vi "数据发送组合-20200825 (子VI).vi"(10 "枚举":T2(ring), 11 "插值后的数组元素":T1) -> (3 "字符串":string)   [LabVIEW 2016, in "数据传输系统-05.lvlib"]
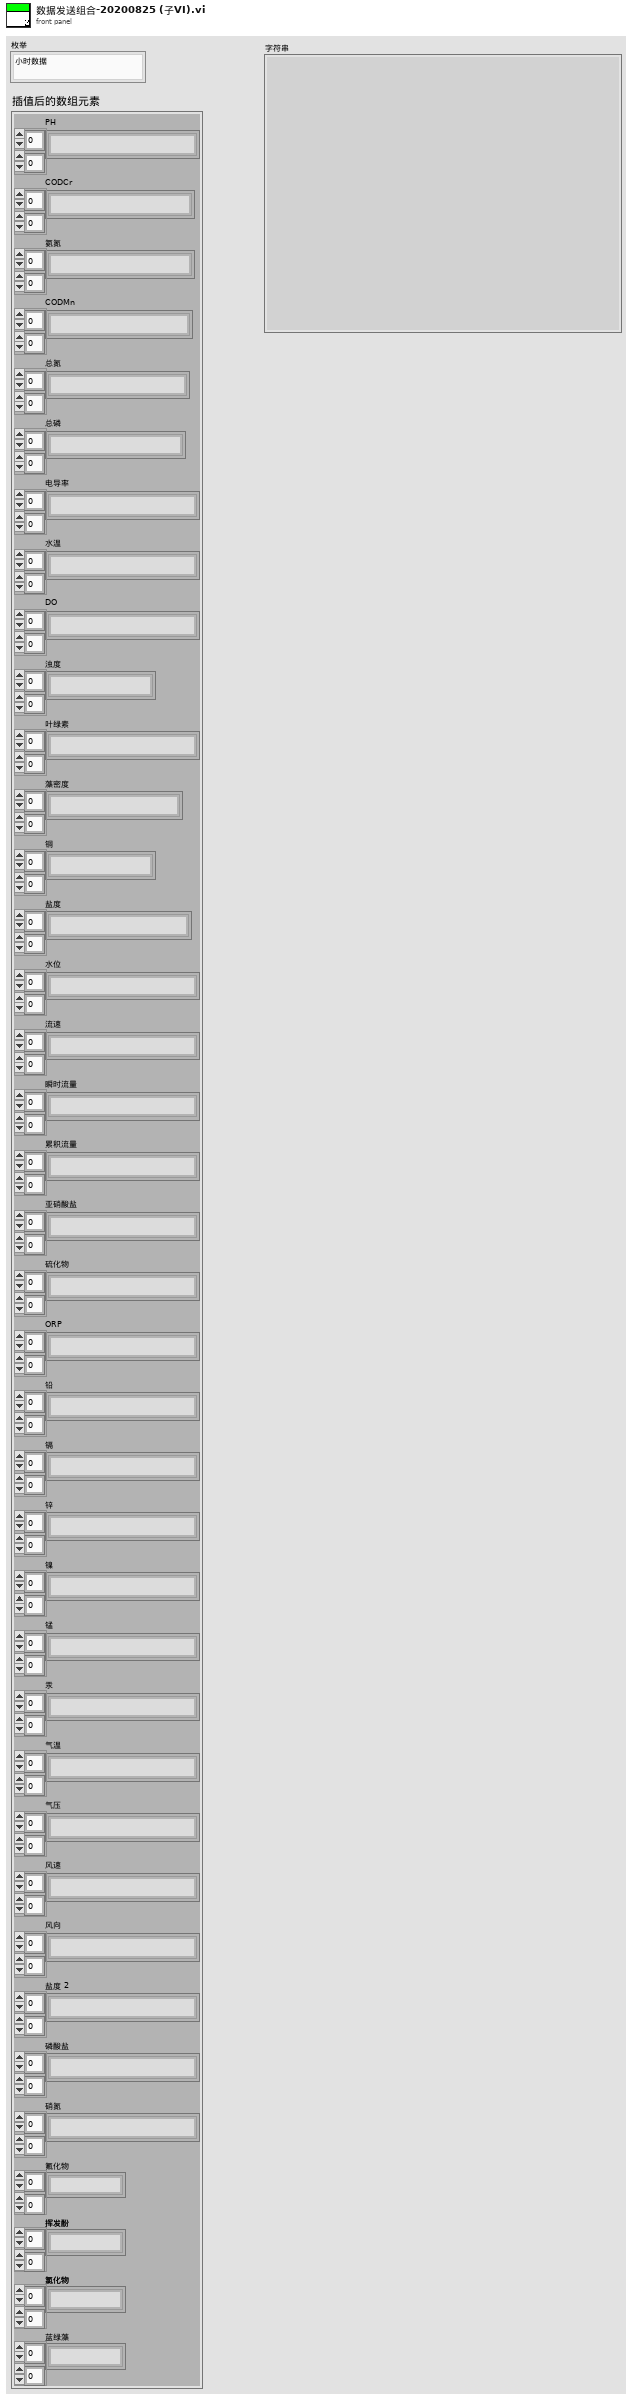
[diagram p1: front panel]
types:
  T1 = cluster{"PH":string[][], "CODCr":string[][], "氨氮":string[][], "CODMn":string[][], "总氮":string[][], "总磷":string[][], "电导率":string[][], "水温":string[][], "DO":string[][], "浊度":string[][], "叶绿素":string[][], "藻密度":string[][], "铜":string[][], "盐度":string[][], "水位":string[][], "流速":string[][], "瞬时流量":string[][], "累积流量":string[][], "亚硝酸盐":string[][], "硫化物":string[][], "ORP":string[][], "铅":string[][], "镉":string[][], "锌":string[][], "镍":string[][], "锰":string[][], "汞":string[][], "气温":string[][], "气压":string[][], "风速":string[][], "风向":string[][], "盐度 2":string[][], "磷酸盐":string[][], "硝氮":string[][], "氟化物":string[][], "挥发酚":string[][], "氯化物":string[][], "蓝绿藻":string[][]}
  T2 = enum16{"小时数据", "实时数据", "平行样测试", "集成干预测试", "加标回收测试", "核查数据", "空白零点跨度数据", "提取小时数据", "提取实时数据", "操作日志", "仪器参数", "3090仪器参数", "提取仪器参数", "报警信息"}
  T3 = cluster{"PH":string[][], "CODCr":string[][], "氨氮":string[][], "CODMn":string[][], "总氮":string[][], "总磷":string[][], "电导率":string[][], "水温":string[][], "DO":string[][], "浊度":string[][], "叶绿素":string[][], "藻密度":string[][], "铜":string[][], "盐度":string[][], "水位":string[][], "流速":string[][], "瞬时流量":string[][], "累积流量":string[][], "亚硝酸盐":string[][], "硫化物":string[][], "ORP":string[][], "铅":string[][], "镉":string[][], "锌":string[][], "镍":string[][], "锰":string[][], "汞":string[][], "气温":string[][], "气压":string[][], "风速":string[][], "风向":string[][], "盐度 2":string[][], "磷酸盐":string[][], "硝氮":string[][], "氟化物":string[][], "挥发酚":string[][], "氯化物":string[][]}
  T4 = cluster{"CODMn":dbl, "CODCr":dbl, "DO":dbl, "铜":dbl, "PH":dbl, "氨氮":dbl, "比电导率":dbl, "水温":dbl, "COD":dbl, "浊度":dbl, "总氮":dbl, "总磷":dbl, "叶绿素a":dbl, "藻密度":dbl, "水位":dbl, "流速":dbl, "瞬时流量":dbl, "累积流量":dbl, "亚硝酸盐":dbl, "硫化物":dbl, "ORP":dbl, "铅":dbl, "镉":dbl, "锌":dbl, "镍":dbl, "锰":dbl, "汞":dbl, "气温":dbl, "气压":dbl, "风速":dbl, "风向":dbl, "盐度":dbl, "磷酸盐":dbl, "硝氮":dbl, "氟化物":dbl, "挥发酚":dbl, "氯化物":dbl, "蓝绿藻":dbl}
  T5 = cluster{"CODMn":string, "CODCr":string, "DO":string, "铜":string, "PH":string, "氨氮":string, "比电导率":string, "水温":string, "COD":string, "浊度":string, "总氮":string, "总磷":string, "叶绿素a":string, "藻密度":string, "水位":string, "流速":string, "瞬时流量":string, "累积流量":string, "亚硝酸盐":string, "硫化物":string, "ORP":string, "铅":string, "镉":string, "锌":string, "镍":string, "锰":string, "汞":string, "气温":string, "气压":string, "风速":string, "风向":string, "盐度":string, "磷酸盐":string, "硝氮":string, "氟化物":string, "挥发酚":string, "氯化物":string, "蓝绿藻":string}
  T6 = typedef "数据传输系统-05.lvlib/应用环境.ctl" = enum16{"STD", "GB212", "婉仪平台"}
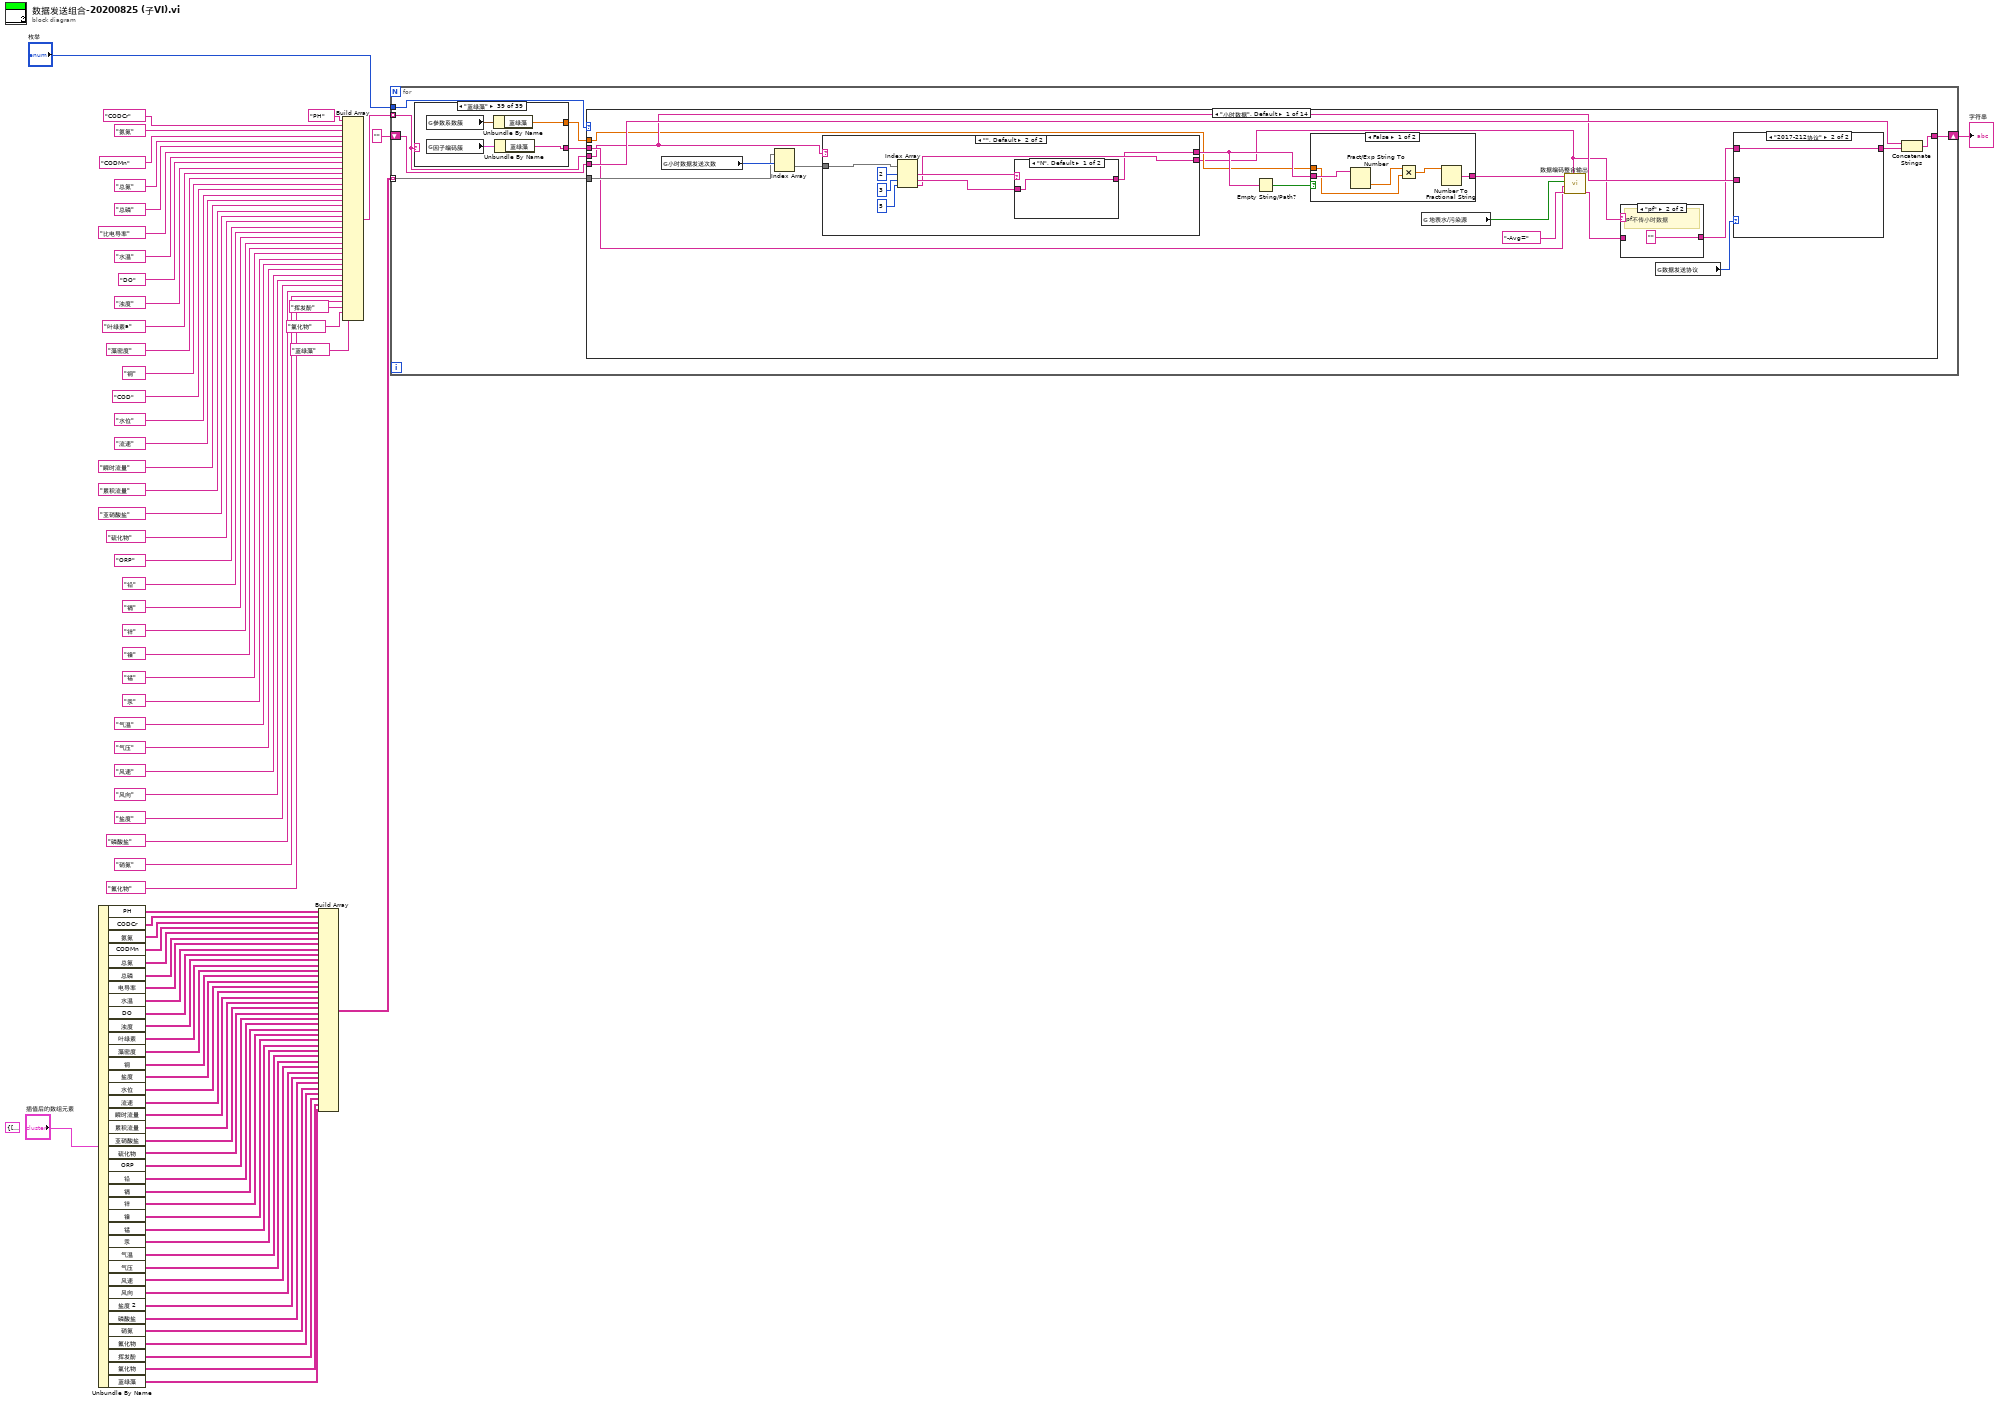
[diagram p0: block diagram]
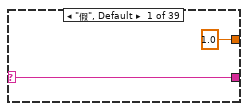
[diagram p2: hidden frame]
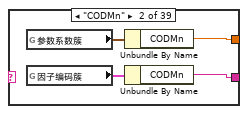
[diagram p3: hidden frame]
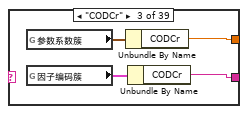
[diagram p4: hidden frame]
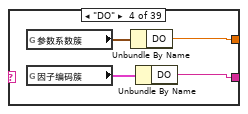
[diagram p5: hidden frame]
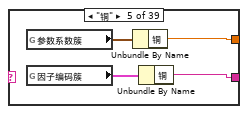
[diagram p6: hidden frame]
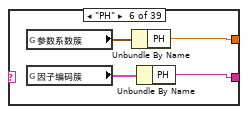
[diagram p7: hidden frame]
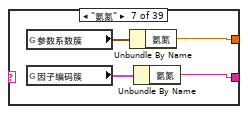
[diagram p8: hidden frame]
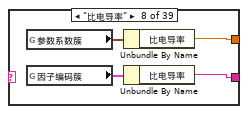
[diagram p9: hidden frame]
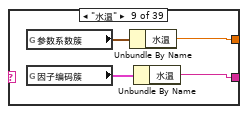
[diagram p10: hidden frame]
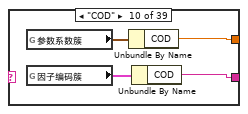
[diagram p11: hidden frame]
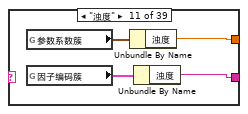
[diagram p12: hidden frame]
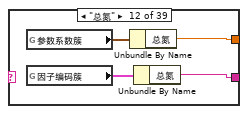
[diagram p13: hidden frame]
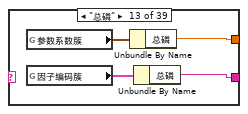
[diagram p14: hidden frame]
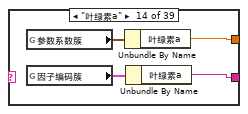
[diagram p15: hidden frame]
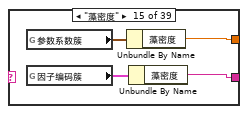
[diagram p16: hidden frame]
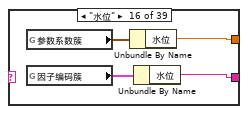
[diagram p17: hidden frame]
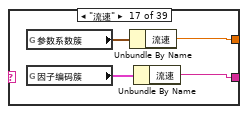
[diagram p18: hidden frame]
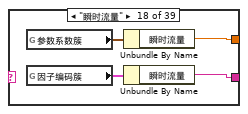
[diagram p19: hidden frame]
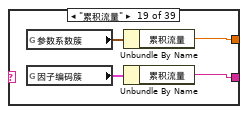
[diagram p20: hidden frame]
diagram:
  (unwired) T3 {"PH"=[], "CODCr"=[], "氨氮"=[], "CODMn"=[], "总氮"=[], "总磷"=[], "电导率"=[], "水温"=[], "DO"=[], "浊度"=[], "叶绿素"=[], "藻密度"=[], "铜"=[], "盐度"=[], "水位"=[], "流速"=[], "瞬时流量"=[], "累积流量"=[], "亚硝酸盐"=[], "硫化物"=[], "ORP"=[], "铅"=[], "镉"=[], "锌"=[], "镍"=[], "锰"=[], "汞"=[], "气温"=[], "气压"=[], "风速"=[], "风向"=[], "盐度 2"=[], "磷酸盐"=[], "硝氮"=[], "氟化物"=[], "挥发酚"=[], "氯化物"=[]} ("插值后的数组元素")
  n1 = Unbundle By Name("插值后的数组元素") -> ("PH"=w82:string[][], "CODCr"=w81:string[][], "氨氮"=w80:string[][], "CODMn"=w79:string[][], "总氮"=w78:string[][], "总磷"=w77:string[][], "电导率"=w76:string[][], "水温"=w75:string[][], "DO"=w74:string[][], "浊度"=w73:string[][], "叶绿素"=w72:string[][], "藻密度"=w71:string[][], "铜"=w70:string[][], "盐度"=w69:string[][], "水位"=w68:string[][], "流速"=w67:string[][], "瞬时流量"=w66:string[][], "累积流量"=w65:string[][], "亚硝酸盐"=w64:string[][], "硫化物"=w63:string[][], "ORP"=w62:string[][], "铅"=w61:string[][], "镉"=w60:string[][], "锌"=w59:string[][], "镍"=w58:string[][], "锰"=w57:string[][], "汞"=w56:string[][], "气温"=w20:string[][], "气压"=w21:string[][], "风速"=w22:string[][], "风向"=w23:string[][], "盐度 2"=w14:string[][], "磷酸盐"=w13:string[][], "硝氮"=w12:string[][], "氟化物"=w8:string[][], "挥发酚"=w6:string[][], "氯化物"=w5:string[][], "蓝绿藻"=w1:string[][])
  n2 = Build Array(w82, w81, w80, w79, w78, w77, w76, w75, w74, w73, w72, w71, w70, w69, w68, w67, w66, w65, w64, w63, w62, w61, w60, w59, w58, w57, w56, w20, w21, w22, w23, w14, w13, w12, w8, w6, w5, w1) -> (w55:string[][][])
  n3 = Build Array("PH" ("污染物编码"), "CODCr" ("污染物编码"), "氨氮" ("污染物编码"), "CODMn" ("污染物编码"), "总氮" ("污染物编码"), "总磷" ("污染物编码"), "比电导率" ("污染物编码"), "水温" ("污染物编码"), "DO" ("污染物编码"), "浊度" ("污染物编码"), "叶绿素a" ("污染物编码"), "藻密度" ("污染物编码"), "铜" ("污染物编码"), "COD" ("污染物编码"), "水位" ("污染物编码"), "流速" ("污染物编码"), "瞬时流量" ("污染物编码"), "累积流量" ("污染物编码"), "亚硝酸盐" ("污染物编码"), "硫化物" ("污染物编码"), "ORP" ("污染物编码"), "铅" ("污染物编码"), "镉" ("污染物编码"), "锌" ("污染物编码"), "镍" ("污染物编码"), "锰" ("污染物编码"), "汞" ("污染物编码"), "气温" ("污染物编码"), "气压" ("污染物编码"), "风速" ("污染物编码"), "风向" ("污染物编码"), "盐度" ("污染物编码"), "磷酸盐" ("污染物编码"), "硝氮" ("污染物编码"), "氟化物" ("污染物编码"), "挥发酚" ("污染物编码"), "氯化物" ("污染物编码"), "蓝绿藻" ("污染物编码")) -> (w27:string[])
  n4 = for {
    tunnel: w55 -> [w89] mode=indexing
    tunnel: w27 -> [w84] mode=indexing
    shift-right: [w88] -> w25
    shift-left: "" -> [w87]
    tunnel: "枚举" -> [w86]
    n5 = case shown="\"蓝绿藻\"" w84 {
      selector: w84 -> [w91 _ _ _ _ _ _ _ _ _ _ _ _ _ _ _ _ _ _ _ _ _ _ _ _ _ _ _ _ _ _ _ _ _ _ _ _ _ _]
      tunnel: [w91 w94 w98 w102 w106 w110 w114 w118 w122 w126 w130 w134 w138 w142 w146 w150 w154 w158 w162 w166 w170 w174 w178 w182 w186 w190 w194 w198 w202 w206 w210 w214 w218 w222 w226 w230 w234 w238 w242] -> w85
      tunnel: [1.0 ("风向") w92 w96 w100 w104 w108 w112 w116 w120 w124 w128 w132 w136 w140 w144 w148 w152 w156 w160 w164 w168 w172 w176 w180 w184 w188 w192 w196 w200 w204 w208 w212 w216 w220 w224 w228 w232 w236 w240] -> w83
      frame "假", Default {
      }
      frame "CODMn" {
        n6 = global read "断电保存全局.vi" "参数系数簇"() -> (w93:T4)
        n7 = global read "断电保存全局.vi" "因子编码簇"() -> (w95:T5)
        n8 = Unbundle By Name(w93) -> ("CODMn"=w92:dbl)
        n9 = Unbundle By Name(w95) -> ("CODMn"=w94:string)
      }
      frame "CODCr" {
        n10 = global read "断电保存全局.vi" "参数系数簇"() -> (w97:T4)
        n11 = global read "断电保存全局.vi" "因子编码簇"() -> (w99:T5)
        n12 = Unbundle By Name(w97) -> ("CODCr"=w96:dbl)
        n13 = Unbundle By Name(w99) -> ("CODCr"=w98:string)
      }
      frame "DO" {
        n14 = global read "断电保存全局.vi" "参数系数簇"() -> (w101:T4)
        n15 = global read "断电保存全局.vi" "因子编码簇"() -> (w103:T5)
        n16 = Unbundle By Name(w101) -> ("DO"=w100:dbl)
        n17 = Unbundle By Name(w103) -> ("DO"=w102:string)
      }
      frame "铜" {
        n18 = global read "断电保存全局.vi" "参数系数簇"() -> (w105:T4)
        n19 = global read "断电保存全局.vi" "因子编码簇"() -> (w107:T5)
        n20 = Unbundle By Name(w105) -> ("铜"=w104:dbl)
        n21 = Unbundle By Name(w107) -> ("铜"=w106:string)
      }
      frame "PH" {
        n22 = global read "断电保存全局.vi" "参数系数簇"() -> (w109:T4)
        n23 = global read "断电保存全局.vi" "因子编码簇"() -> (w111:T5)
        n24 = Unbundle By Name(w109) -> ("PH"=w108:dbl)
        n25 = Unbundle By Name(w111) -> ("PH"=w110:string)
      }
      frame "氨氮" {
        n26 = global read "断电保存全局.vi" "参数系数簇"() -> (w113:T4)
        n27 = global read "断电保存全局.vi" "因子编码簇"() -> (w115:T5)
        n28 = Unbundle By Name(w113) -> ("氨氮"=w112:dbl)
        n29 = Unbundle By Name(w115) -> ("氨氮"=w114:string)
      }
      frame "比电导率" {
        n30 = global read "断电保存全局.vi" "参数系数簇"() -> (w117:T4)
        n31 = global read "断电保存全局.vi" "因子编码簇"() -> (w119:T5)
        n32 = Unbundle By Name(w117) -> ("比电导率"=w116:dbl)
        n33 = Unbundle By Name(w119) -> ("比电导率"=w118:string)
      }
      frame "水温" {
        n34 = global read "断电保存全局.vi" "参数系数簇"() -> (w121:T4)
        n35 = global read "断电保存全局.vi" "因子编码簇"() -> (w123:T5)
        n36 = Unbundle By Name(w121) -> ("水温"=w120:dbl)
        n37 = Unbundle By Name(w123) -> ("水温"=w122:string)
      }
      frame "COD" {
        n38 = global read "断电保存全局.vi" "参数系数簇"() -> (w125:T4)
        n39 = global read "断电保存全局.vi" "因子编码簇"() -> (w127:T5)
        n40 = Unbundle By Name(w125) -> ("COD"=w124:dbl)
        n41 = Unbundle By Name(w127) -> ("COD"=w126:string)
      }
      frame "浊度" {
        n42 = global read "断电保存全局.vi" "参数系数簇"() -> (w129:T4)
        n43 = global read "断电保存全局.vi" "因子编码簇"() -> (w131:T5)
        n44 = Unbundle By Name(w129) -> ("浊度"=w128:dbl)
        n45 = Unbundle By Name(w131) -> ("浊度"=w130:string)
      }
      frame "总氮" {
        n46 = global read "断电保存全局.vi" "参数系数簇"() -> (w133:T4)
        n47 = global read "断电保存全局.vi" "因子编码簇"() -> (w135:T5)
        n48 = Unbundle By Name(w133) -> ("总氮"=w132:dbl)
        n49 = Unbundle By Name(w135) -> ("总氮"=w134:string)
      }
      frame "总磷" {
        n50 = global read "断电保存全局.vi" "参数系数簇"() -> (w137:T4)
        n51 = global read "断电保存全局.vi" "因子编码簇"() -> (w139:T5)
        n52 = Unbundle By Name(w137) -> ("总磷"=w136:dbl)
        n53 = Unbundle By Name(w139) -> ("总磷"=w138:string)
      }
      frame "叶绿素a" {
        n54 = global read "断电保存全局.vi" "参数系数簇"() -> (w141:T4)
        n55 = global read "断电保存全局.vi" "因子编码簇"() -> (w143:T5)
        n56 = Unbundle By Name(w141) -> ("叶绿素a"=w140:dbl)
        n57 = Unbundle By Name(w143) -> ("叶绿素a"=w142:string)
      }
      frame "藻密度" {
        n58 = global read "断电保存全局.vi" "参数系数簇"() -> (w145:T4)
        n59 = global read "断电保存全局.vi" "因子编码簇"() -> (w147:T5)
        n60 = Unbundle By Name(w145) -> ("藻密度"=w144:dbl)
        n61 = Unbundle By Name(w147) -> ("藻密度"=w146:string)
      }
      frame "水位" {
        n62 = global read "断电保存全局.vi" "参数系数簇"() -> (w149:T4)
        n63 = global read "断电保存全局.vi" "因子编码簇"() -> (w151:T5)
        n64 = Unbundle By Name(w149) -> ("水位"=w148:dbl)
        n65 = Unbundle By Name(w151) -> ("水位"=w150:string)
      }
      frame "流速" {
        n66 = global read "断电保存全局.vi" "参数系数簇"() -> (w153:T4)
        n67 = global read "断电保存全局.vi" "因子编码簇"() -> (w155:T5)
        n68 = Unbundle By Name(w153) -> ("流速"=w152:dbl)
        n69 = Unbundle By Name(w155) -> ("流速"=w154:string)
      }
      frame "瞬时流量" {
        n70 = global read "断电保存全局.vi" "参数系数簇"() -> (w157:T4)
        n71 = global read "断电保存全局.vi" "因子编码簇"() -> (w159:T5)
        n72 = Unbundle By Name(w157) -> ("瞬时流量"=w156:dbl)
        n73 = Unbundle By Name(w159) -> ("瞬时流量"=w158:string)
      }
      frame "累积流量" {
        n74 = global read "断电保存全局.vi" "参数系数簇"() -> (w161:T4)
        n75 = global read "断电保存全局.vi" "因子编码簇"() -> (w163:T5)
        n76 = Unbundle By Name(w161) -> ("累积流量"=w160:dbl)
        n77 = Unbundle By Name(w163) -> ("累积流量"=w162:string)
      }
      frame "亚硝酸盐" {
        n78 = global read "断电保存全局.vi" "参数系数簇"() -> (w165:T4)
        n79 = global read "断电保存全局.vi" "因子编码簇"() -> (w167:T5)
        n80 = Unbundle By Name(w165) -> ("亚硝酸盐"=w164:dbl)
        n81 = Unbundle By Name(w167) -> ("亚硝酸盐"=w166:string)
      }
      frame "硫化物" {
        n82 = global read "断电保存全局.vi" "参数系数簇"() -> (w169:T4)
        n83 = global read "断电保存全局.vi" "因子编码簇"() -> (w171:T5)
        n84 = Unbundle By Name(w169) -> ("硫化物"=w168:dbl)
        n85 = Unbundle By Name(w171) -> ("硫化物"=w170:string)
      }
      frame "ORP" {
        n86 = global read "断电保存全局.vi" "参数系数簇"() -> (w173:T4)
        n87 = global read "断电保存全局.vi" "因子编码簇"() -> (w175:T5)
        n88 = Unbundle By Name(w173) -> ("ORP"=w172:dbl)
        n89 = Unbundle By Name(w175) -> ("ORP"=w174:string)
      }
      frame "铅" {
        n90 = global read "断电保存全局.vi" "参数系数簇"() -> (w177:T4)
        n91 = global read "断电保存全局.vi" "因子编码簇"() -> (w179:T5)
        n92 = Unbundle By Name(w177) -> ("铅"=w176:dbl)
        n93 = Unbundle By Name(w179) -> ("铅"=w178:string)
      }
      frame "镉" {
        n94 = global read "断电保存全局.vi" "参数系数簇"() -> (w181:T4)
        n95 = global read "断电保存全局.vi" "因子编码簇"() -> (w183:T5)
        n96 = Unbundle By Name(w181) -> ("镉"=w180:dbl)
        n97 = Unbundle By Name(w183) -> ("镉"=w182:string)
      }
      frame "锌" {
        n98 = global read "断电保存全局.vi" "参数系数簇"() -> (w185:T4)
        n99 = global read "断电保存全局.vi" "因子编码簇"() -> (w187:T5)
        n100 = Unbundle By Name(w185) -> ("锌"=w184:dbl)
        n101 = Unbundle By Name(w187) -> ("锌"=w186:string)
      }
      frame "镍" {
        n102 = global read "断电保存全局.vi" "参数系数簇"() -> (w189:T4)
        n103 = global read "断电保存全局.vi" "因子编码簇"() -> (w191:T5)
        n104 = Unbundle By Name(w189) -> ("镍"=w188:dbl)
        n105 = Unbundle By Name(w191) -> ("镍"=w190:string)
      }
      frame "锰" {
        n106 = global read "断电保存全局.vi" "参数系数簇"() -> (w193:T4)
        n107 = global read "断电保存全局.vi" "因子编码簇"() -> (w195:T5)
        n108 = Unbundle By Name(w193) -> ("锰"=w192:dbl)
        n109 = Unbundle By Name(w195) -> ("锰"=w194:string)
      }
      frame "汞" {
        n110 = global read "断电保存全局.vi" "参数系数簇"() -> (w197:T4)
        n111 = global read "断电保存全局.vi" "因子编码簇"() -> (w199:T5)
        n112 = Unbundle By Name(w197) -> ("汞"=w196:dbl)
        n113 = Unbundle By Name(w199) -> ("汞"=w198:string)
      }
      frame "气温" {
        n114 = global read "断电保存全局.vi" "参数系数簇"() -> (w201:T4)
        n115 = global read "断电保存全局.vi" "因子编码簇"() -> (w203:T5)
        n116 = Unbundle By Name(w201) -> ("气温"=w200:dbl)
        n117 = Unbundle By Name(w203) -> ("气温"=w202:string)
      }
      frame "气压" {
        n118 = global read "断电保存全局.vi" "参数系数簇"() -> (w205:T4)
        n119 = global read "断电保存全局.vi" "因子编码簇"() -> (w207:T5)
        n120 = Unbundle By Name(w205) -> ("气压"=w204:dbl)
        n121 = Unbundle By Name(w207) -> ("气压"=w206:string)
      }
      frame "风速" {
        n122 = global read "断电保存全局.vi" "参数系数簇"() -> (w209:T4)
        n123 = global read "断电保存全局.vi" "因子编码簇"() -> (w211:T5)
        n124 = Unbundle By Name(w209) -> ("风速"=w208:dbl)
        n125 = Unbundle By Name(w211) -> ("风速"=w210:string)
      }
      frame "风向" {
        n126 = global read "断电保存全局.vi" "参数系数簇"() -> (w213:T4)
        n127 = global read "断电保存全局.vi" "因子编码簇"() -> (w215:T5)
        n128 = Unbundle By Name(w213) -> ("风向"=w212:dbl)
        n129 = Unbundle By Name(w215) -> ("风向"=w214:string)
      }
      frame "盐度" {
        n130 = global read "断电保存全局.vi" "参数系数簇"() -> (w217:T4)
        n131 = global read "断电保存全局.vi" "因子编码簇"() -> (w219:T5)
        n132 = Unbundle By Name(w217) -> ("盐度"=w216:dbl)
        n133 = Unbundle By Name(w219) -> ("盐度"=w218:string)
      }
      frame "磷酸盐" {
        n134 = global read "断电保存全局.vi" "参数系数簇"() -> (w221:T4)
        n135 = global read "断电保存全局.vi" "因子编码簇"() -> (w223:T5)
        n136 = Unbundle By Name(w221) -> ("磷酸盐"=w220:dbl)
        n137 = Unbundle By Name(w223) -> ("磷酸盐"=w222:string)
      }
      frame "硝氮" {
        n138 = global read "断电保存全局.vi" "参数系数簇"() -> (w225:T4)
        n139 = global read "断电保存全局.vi" "因子编码簇"() -> (w227:T5)
        n140 = Unbundle By Name(w225) -> ("硝氮"=w224:dbl)
        n141 = Unbundle By Name(w227) -> ("硝氮"=w226:string)
      }
      frame "氟化物" {
        n142 = global read "断电保存全局.vi" "参数系数簇"() -> (w229:T4)
        n143 = global read "断电保存全局.vi" "因子编码簇"() -> (w231:T5)
        n144 = Unbundle By Name(w229) -> ("氟化物"=w228:dbl)
        n145 = Unbundle By Name(w231) -> ("氟化物"=w230:string)
      }
      frame "挥发酚" {
        n146 = global read "断电保存全局.vi" "参数系数簇"() -> (w233:T4)
        n147 = global read "断电保存全局.vi" "因子编码簇"() -> (w235:T5)
        n148 = Unbundle By Name(w233) -> ("挥发酚"=w232:dbl)
        n149 = Unbundle By Name(w235) -> ("挥发酚"=w234:string)
      }
      frame "氯化物" {
        n150 = global read "断电保存全局.vi" "参数系数簇"() -> (w237:T4)
        n151 = global read "断电保存全局.vi" "因子编码簇"() -> (w239:T5)
        n152 = Unbundle By Name(w237) -> ("氯化物"=w236:dbl)
        n153 = Unbundle By Name(w239) -> ("氯化物"=w238:string)
      }
      frame "蓝绿藻" {
        n154 = global read "断电保存全局.vi" "参数系数簇"() -> (w241:T4)
        n155 = global read "断电保存全局.vi" "因子编码簇"() -> (w243:T5)
        n156 = Unbundle By Name(w241) -> ("蓝绿藻"=w240:dbl)
        n157 = Unbundle By Name(w243) -> ("蓝绿藻"=w242:string)
      }
    }
    n158 = case shown="\"小时数据\", Default" w86 {
      tunnel: w89 -> [w258 w303 w334 w343 w398 w404 w416 w440 w462 w499 w517 w524 w534 w556]
      tunnel: w85 -> [w254 w296 w333 w344 w394 w403 w415 w434 w461 w487 w515 w522 w533 w559]
      tunnel: [w257 w300 w335 w341 w399 w400 w412 w431 w460 w494 w512 w521 w529 w545] -> w88
      tunnel: w87 -> [w256 w301 w337 w342 w395 w402 w413 w432 w463 w495 w513 w523 w530 w540]
      tunnel: w84 -> [w252 w295 _ w338 _ _ _ _ _ _ _ _ _ w554]
      tunnel: w83 -> [w249 w291 _ w339 _ _ _ w427 w456 _ _ _ _ _]
      frame "小时数据", Default {
        n159 = global read "全局 小时数据发送次数.vi" "小时数据发送次数"() -> (w261:i32)
        n160 = Index Array(array=w258, index (row)=w261) -> (element=w260:string[])  [unwired: 1 in]
        n161 = case shown="\"\", Default" w252 {
          tunnel: w260 -> [w273 w276]
          tunnel: [w270 w274] -> w250
          tunnel: ["N" ("字符串") w275] -> w246
          frame "风速", "风向", "累积流量", "流速", "气温", "气压", "水位", "瞬时流量" {
            n162 = Index Array(array=w273, index=1 ("索引")) -> (element=w270:string)
          }
          frame "", Default {
            n163 = Index Array(array=w276, index #1=2 ("索引"), index #2=3 ("索引"), index #3=5 ("索引")) -> (element #1=w279:string, element #2=w278:string, element #3=w275:string)
            n164 = case shown="\"N\", Default" w279 {
              tunnel: [w282 ""] -> w274
              tunnel: w278 -> [w282 _]
              frame "N", Default {
              }
              frame "M" {
              }
            }
          }
        }
        n165 = Empty String/Path?(string/path=w250) -> (empty?=w251:bool)
        n166 = case shown="False" w251 {
          tunnel: w250 -> [w267 w269]
          tunnel: w249 -> [w266 _]
          tunnel: [w264 w269] -> w248
          frame False {
            n167 = Fract/Exp String To Number(string=w267) -> (number=w268:dbl)  [unwired: 3 in, 1 out]
            n168 = Multiply(x=w268, y=w266) -> (x*y=w265:dbl)
            n169 = Number To Fractional String(number=w265) -> (F-format string=w264:string)  [unwired: 3 in]
          }
          frame True {
            # "空"
          }
        }
        n170 = global read "断电保存全局.vi" "地表水/污染源"() -> (w247:bool)
        n171 = call "数据编码整合输出.vi"("数据标识"=w246, "数据类型"="-Avg=", "污染物编码"=w254, "地表水/污染源"=w247, "数据值"=w248) -> ("编码输出"=w245:string)  [unwired: 6 in]
        n172 = case shown="\"pf\"" w246 {
          tunnel: w245 -> [w262 _]
          tunnel: [w262 ""] -> w244
          frame "假", Default {
          }
          frame "pf" {
            # "pf不传小时数据"
          }
        }
        n173 = global read "断电保存全局.vi" "数据发送协议"() -> (w255:enum16{"2005-212协议", "2017-212协议"})
        n174 = case shown="\"2017-212协议\"" w255 {
          tunnel: w252 -> [w286 _]
          tunnel: w244 -> [w284 w289]
          tunnel: [w285 w289] -> w253
          frame "2005-212协议", Default {
            n175 = case shown="\"风速\", \"风向\", \"累积流量\", \"流速\", \"气温\", \"气压\", \"水位\"" w286 {
              tunnel: [w287 ""] -> w285
              tunnel: w284 -> [w287 _]
              frame "假", Default {
              }
              frame "风速", "风向", "累积流量", "流速", "气温", "气压", "水位" {
              }
            }
          }
          frame "2017-212协议" {
          }
        }
        n176 = Concatenate Strings(w256, w253) -> (w257:string)
      }
      frame "实时数据" {
        n177 = global read "全局 小时数据发送次数.vi" "小时数据发送次数"() -> (w304:i32)
        n178 = Index Array(array=w303, index (row)=w304) -> (element=w305:string[])  [unwired: 1 in]
        n179 = case shown="\"\", Default" w295 {
          tunnel: w305 -> [w314 w318 w324]
          tunnel: [w313 w317 w323] -> w293
          tunnel: ["N" ("字符串") "N" ("字符串") w321] -> w302
          frame "累积流量", "流速", "水位", "瞬时流量" {
            n180 = Index Array(array=w314, index=1 ("索引")) -> (element=w313:string)
          }
          frame "风速", "风向", "气温", "气压" {
            n181 = Index Array(array=w318, index=1 ("索引")) -> (element=w317:string)
          }
          frame "", Default {
            n182 = Index Array(array=w324, index #1=3 ("索引"), index #2=5 ("索引")) -> (element #1=w323:string, element #2=w321:string)
          }
        }
        n183 = Empty String/Path?(string/path=w293) -> (empty?=w294:bool)
        n184 = case shown="False" w294 {
          tunnel: w293 -> [w310 w312]
          tunnel: w291 -> [w309 _]
          tunnel: [w307 w312] -> w292
          frame False {
            n185 = Fract/Exp String To Number(string=w310) -> (number=w311:dbl)  [unwired: 3 in, 1 out]
            n186 = Multiply(x=w311, y=w309) -> (x*y=w308:dbl)
            n187 = Number To Fractional String(number=w308) -> (F-format string=w307:string)  [unwired: 3 in]
          }
          frame True {
            # "空"
          }
        }
        n188 = global read "断电保存全局.vi" "数据发送协议"() -> (w299:enum16{"2005-212协议", "2017-212协议"})
        n189 = call "数据编码整合输出.vi"("数据标识"=w302, "数据类型"="-Rtd=", "污染物编码"=w296, "地表水/污染源"=FALSE, "数据值"=w292) -> ("编码输出"=w298:string)  [unwired: 6 in]
        n190 = case shown="\"2017-212协议\"" w299 {
          tunnel: w295 -> [w328 _]
          tunnel: w298 -> [w326 w331]
          tunnel: [w327 w331] -> w297
          frame "2005-212协议", Default {
            n191 = case shown="\"假\", Default" w328 {
              tunnel: [w329 ""] -> w327
              tunnel: w326 -> [w329 _]
              frame "假", Default {
              }
              frame "风速", "风向", "累积流量", "流速", "气温", "气压", "水位" {
              }
            }
          }
          frame "2017-212协议" {
          }
        }
        n192 = Concatenate Strings(w301, w297) -> (w300:string)
      }
      frame "平行样测试" {
        n193 = global read "全局 小时数据发送次数.vi" "小时数据发送次数"() -> (w332:i32)
        n194 = call "平行样集成干预数据组合(子VI).vi"("污染物编码"=w333, "数据输入"=w334, "小时数据发送次数"=w332) -> ("输出组合"=w336:string)  [unwired: 8 in]
        n195 = Concatenate Strings(w337, w336) -> (w335:string)
      }
      frame "集成干预测试" {
        n196 = global read "断电保存全局.vi" "应用环境"() -> (w340:T6)
        n197 = case shown="\"GB212\", Default" w340 {
          tunnel: w344 -> [w348 w354]
          tunnel: w343 -> [w347 w355]
          tunnel: w342 -> [w346 w356]
          tunnel: [w345 w351] -> w341
          tunnel: w339 -> [_ w353]
          tunnel: w338 -> [_ w352]
          frame "STD" {
            n198 = global read "全局 小时数据发送次数.vi" "小时数据发送次数"() -> (w349:i32)
            n199 = call "平行样集成干预数据组合(子VI).vi"("污染物编码"=w348, "数据输入"=w347, "小时数据发送次数"=w349) -> ("输出组合"=w350:string)  [unwired: 8 in]
            n200 = Concatenate Strings(w346, w350) -> (w345:string)
          }
          frame "GB212", Default {
            n201 = global read "全局 小时数据发送次数.vi" "小时数据发送次数"() -> (w367:i32)
            n202 = Index Array(array=w355, index (row)=w367) -> (element=w366:string[])  [unwired: 1 in]
            n203 = case shown="\"\", Default" w352 {
              tunnel: w366 -> [w377 w380]
              tunnel: [w374 w379] -> w359
              tunnel: ["N" ("字符串") w378] -> w364
              frame "风速", "风向", "累积流量", "流速", "气温", "气压", "水位", "瞬时流量" {
                n204 = Index Array(array=w377, index=1 ("索引")) -> (element=w374:string)
              }
              frame "", Default {
                n205 = Index Array(array=w380, index #1=2 ("索引"), index #2=3 ("索引"), index #3=5 ("索引")) -> (element #1=w383:string, element #2=w382:string, element #3=w378:string)
                n206 = case shown="\"N\", Default" w383 {
                  tunnel: [w386 ""] -> w379
                  tunnel: w382 -> [w386 _]
                  frame "N", Default {
                  }
                  frame "M" {
                  }
                }
              }
            }
            n207 = Empty String/Path?(string/path=w359) -> (empty?=w360:bool)
            n208 = case shown="False" w360 {
              tunnel: w359 -> [w371 w373]
              tunnel: w353 -> [w370 _]
              tunnel: [w368 w373] -> w358
              frame False {
                n209 = Fract/Exp String To Number(string=w371) -> (number=w372:dbl)  [unwired: 3 in, 1 out]
                n210 = Multiply(x=w372, y=w370) -> (x*y=w369:dbl)
                n211 = Number To Fractional String(number=w369) -> (F-format string=w368:string)  [unwired: 3 in]
              }
              frame True {
                # "空"
              }
            }
            n212 = global read "断电保存全局.vi" "地表水/污染源"() -> (w357:bool)
            n213 = global read "断电保存全局.vi" "数据发送协议"() -> (w363:enum16{"2005-212协议", "2017-212协议"})
            n214 = call "数据编码整合输出.vi"("数据标识"=w364, "数据类型"="-Avg=", "污染物编码"=w354, "地表水/污染源"=w357, "数据值"=w358) -> ("编码输出"=w362:string)  [unwired: 6 in]
            n215 = case shown="\"2017-212协议\"" w363 {
              tunnel: w352 -> [w390 _]
              tunnel: w362 -> [w388 w393]
              tunnel: [w389 w393] -> w361
              frame "2005-212协议", Default {
                n216 = case shown="\"假\", Default" w390 {
                  tunnel: [w391 ""] -> w389
                  tunnel: w388 -> [w391 _]
                  frame "假", Default {
                  }
                  frame "风速", "风向", "累积流量", "流速", "气温", "气压", "水位" {
                  }
                }
              }
              frame "2017-212协议" {
              }
            }
            n217 = Concatenate Strings(w356, w361) -> (w351:string)
          }
        }
      }
      frame "加标回收测试" {
        n218 = global read "全局 小时数据发送次数.vi" "小时数据发送次数"() -> (w397:i32)
        n219 = call "加标回收数据组合 (子VI).vi"("小时数据发送次数"=w397, "数据"=w398, "污染物编码"=w394) -> ("组合输出"=w396:string)  [unwired: 7 in, 1 out]
        n220 = Concatenate Strings(w395, w396) -> (w399:string)
      }
      frame "核查数据" {
        n221 = global read "全局 小时数据发送次数.vi" "小时数据发送次数"() -> (w405:i32)
        n222 = call "标样核查数据组合(子VI).vi"("小时数据发送次数"=w405, "数据输入"=w404, "污染物编码"=w403) -> ("输出组合"=w401:string)  [unwired: 8 in]
        n223 = Concatenate Strings(w402, w401) -> (w400:string)
      }
      frame "空白零点跨度数据" {
        n224 = global read "全局 小时数据发送次数.vi" "小时数据发送次数"() -> (w418:i32)
        n225 = Index Array(array=w416, index (row)=w418) -> (element=w422:string[])  [unwired: 1 in]
        n226 = Index Array(array=w422, index #1=0 ("索引"), index #2=3 ("索引"), index #3=6 ("索引"), index #4=7 ("索引"), index #5=5 ("索引")) -> (element #2=w417:string, element #3=w419:string, element #4=w408:string, element #5=w406:string)  [unwired: 1 out]
        n227 = Empty String/Path?(string/path=w408) -> (empty?=w410:bool)
        n228 = case shown="False" w410 {
          tunnel: [w424 "0" ("span value")] -> w409
          tunnel: w408 -> [w424 _]
          frame False {
          }
          frame True {
          }
        }
        n229 = call "零点跨度数据组合 (子VI).vi"("数据标识"=w406, "span value"=w409, "standard value"=w419, "check value"=w417, "污染物编码"=w415) -> ("组合输出"=w414:string)  [unwired: 6 in]
        n230 = Concatenate Strings(w413, w414) -> (w412:string)
      }
      frame "提取小时数据" {
        n231 = global read "全局 小时数据发送次数.vi" "小时数据发送次数"() -> (w441:i32)
        n232 = Index Array(array=w440, index (row)=w441) -> (element=w439:string[])  [unwired: 1 in]
        n233 = Index Array(array=w439, index #2=1 ("索引")) -> (element #2=w428:string)  [unwired: 1 in, 1 out]
        n234 = Empty String/Path?(string/path=w428) -> (empty?=w430:bool)
        n235 = case shown="False" w430 {
          tunnel: w428 -> [w446 w448]
          tunnel: w427 -> [w445 _]
          tunnel: [w443 w448] -> w429
          frame False {
            n236 = Fract/Exp String To Number(string=w446) -> (number=w447:dbl)  [unwired: 3 in, 1 out]
            n237 = Multiply(x=w447, y=w445) -> (x*y=w444:dbl)
            n238 = Number To Fractional String(number=w444) -> (F-format string=w443:string)  [unwired: 3 in]
          }
          frame True {
            # "空"
          }
        }
        n239 = global read "断电保存全局.vi" "地表水/污染源"() -> (w426:bool)
        n240 = global read "断电保存全局.vi" "数据发送协议"() -> (w436:enum16{"2005-212协议", "2017-212协议"})
        n241 = call "数据编码整合输出.vi"("数据标识"="N", "数据类型"="-Avg=", "污染物编码"=w434, "地表水/污染源"=w426, "数据值"=w429) -> ("编码输出"=w433:string)  [unwired: 6 in]
        n242 = case shown="\"2005-212协议\", Default" w436 {
          tunnel: w434 -> [w451 _]
          tunnel: w433 -> [w449 w454]
          tunnel: [w450 w454] -> w435
          frame "2005-212协议", Default {
            n243 = case shown="\"假\", Default" w451 {
              tunnel: [w452 ""] -> w450
              tunnel: w449 -> [w452 _]
              frame "假", Default {
              }
              frame "累积流量", "流速", "水位" {
              }
            }
          }
          frame "2017-212协议" {
          }
        }
        n244 = Concatenate Strings(w432, w435) -> (w431:string)
      }
      frame "提取实时数据" {
        n245 = global read "全局 小时数据发送次数.vi" "小时数据发送次数"() -> (w469:i32)
        n246 = Index Array(array=w462, index (row)=w469) -> (element=w470:string[])  [unwired: 1 in]
        n247 = Index Array(array=w470, index #1=3 ("索引"), index #2=5 ("索引")) -> (element #1=w457:string, element #2=w467:string)
        n248 = Empty String/Path?(string/path=w457) -> (empty?=w459:bool)
        n249 = case shown="False" w459 {
          tunnel: w457 -> [w476 w478]
          tunnel: w456 -> [w475 _]
          tunnel: [w473 w478] -> w458
          frame False {
            n250 = Fract/Exp String To Number(string=w476) -> (number=w477:dbl)  [unwired: 3 in, 1 out]
            n251 = Multiply(x=w477, y=w475) -> (x*y=w474:dbl)
            n252 = Number To Fractional String(number=w474) -> (F-format string=w473:string)  [unwired: 3 in]
          }
          frame True {
            # "空"
          }
        }
        n253 = global read "断电保存全局.vi" "地表水/污染源"() -> (w455:bool)
        n254 = global read "断电保存全局.vi" "数据发送协议"() -> (w466:enum16{"2005-212协议", "2017-212协议"})
        n255 = call "数据编码整合输出.vi"("数据标识"=w467, "数据类型"="-Rtd=", "污染物编码"=w461, "地表水/污染源"=w455, "数据值"=w458) -> ("编码输出"=w465:string)  [unwired: 6 in]
        n256 = case shown="\"2017-212协议\"" w466 {
          tunnel: w461 -> [w481 _]
          tunnel: w465 -> [w479 w484]
          tunnel: [w480 w484] -> w464
          frame "2005-212协议", Default {
            n257 = case shown="\"累积流量\", \"流速\", \"水位\"" w481 {
              tunnel: [w482 ""] -> w480
              tunnel: w479 -> [w482 _]
              frame "假", Default {
              }
              frame "累积流量", "流速", "水位" {
              }
            }
          }
          frame "2017-212协议" {
          }
        }
        n258 = Concatenate Strings(w463, w464) -> (w460:string)
      }
      frame "操作日志" {
        n259 = global read "断电保存全局.vi" "因子编码簇"() -> (w490:T5)
        n260 = global read "全局 小时数据发送次数.vi" "小时数据发送次数"() -> (w503:i32)
        n261 = Unbundle By Name(w490) -> ("DO"=w489:string)
        n262 = Equal?(x=w487, y=w489) -> (x = y?=w485:bool)
        n263 = Index Array(array=w499, index (row)=w503) -> (element=w498:string[])  [unwired: 1 in]
        n264 = Index Array(array=w498, index #1=0 ("索引"), index #2=2 ("索引")) -> (element #2=w497:string)  [unwired: 1 out]
        n265 = Empty String/Path?(string/path=w497) -> (empty?=w502:bool)
        n266 = Select(t="w00000", s=w485, f=w487) -> (s? t:f=w486:string)
        n267 = Select(t="i21001", s=w485, f="i11001") -> (s? t:f=w491:string)
        n268 = case shown="False" w502 {
          tunnel: [w507 ""] -> w496
          tunnel: w497 -> [w505 _]
          tunnel: w486 -> [w506 _]
          tunnel: w491 -> [w504 _]
          frame False {
            n269 = Format Into String(format string="PolId=%s,%s-Info=//%s//;" ("格式字符串"), w506, w504, w505) -> (resulting string=w507:string)  [unwired: 2 in, 1 out]
          }
          frame True {
          }
        }
        n270 = Concatenate Strings(w495, w496) -> (w494:string)
      }
      frame "仪器参数" {
        n271 = global read "断电保存全局.vi" "应用环境"() -> (w511:T6)
        n272 = global read "全局 小时数据发送次数.vi" "小时数据发送次数"() -> (w518:i32)
        n273 = case shown="\"GB212\", Default" w511 {
          tunnel: ["3090仪器参数" ("table") "仪器参数" ("table")] -> w510
          frame "STD" {
          }
          frame "GB212", Default {
          }
        }
        n274 = Index Array(array=w517, index (row)=w518) -> (element=w516:string[])  [unwired: 1 in]
        n275 = call "关键参数组合 (子VI).vi"("table"=w510, "因子编码"=w515, "data"=w516) -> ("字符串"=w514:string)  [unwired: 8 in]
        n276 = Concatenate Strings(w513, w514) -> (w512:string)
      }
      frame "3090仪器参数" {
        n277 = global read "全局 小时数据发送次数.vi" "小时数据发送次数"() -> (w528:i32)
        n278 = Index Array(array=w524, index (row)=w528) -> (element=w526:string[])  [unwired: 1 in]
        n279 = call "关键参数组合 (子VI).vi"("table"="3090仪器参数", "因子编码"=w522, "data"=w526) -> ("字符串"=w525:string)  [unwired: 8 in]
        n280 = Concatenate Strings(w523, w525) -> (w521:string)
      }
      frame "提取仪器参数" {
        n281 = global read "全局 小时数据发送次数.vi" "小时数据发送次数"() -> (w535:i32)
        n282 = Index Array(array=w534, index (row)=w535) -> (element=w532:string[])  [unwired: 1 in]
        n283 = call "提取仪器参数 (子VI).vi"("因子编码"=w533, "数据输入"=w532) -> ("字符串"=w531:string)  [unwired: 9 in]
        n284 = Concatenate Strings(w530, w531) -> (w529:string)
      }
      frame "报警信息" {
        n285 = Empty String/Path?(string/path=w540) -> (empty?=w539:bool)
        n286 = global read "断电保存全局.vi" "因子编码簇"() -> (w562:T5)
        n287 = case shown="\"CODMn\"" w554 {
          tunnel: [u16 0 ("register") w580 w586 w592 w598 w604] -> w552
          tunnel: [u16 0 ("register") w577 w583 w589 w595 w601] -> w537
          frame "假", Default {
          }
          frame "CODMn" {
            n288 = global read "全局1.vi" "读取试剂余量的值"() -> (w578:u16[])
            n289 = global read "全局1.vi" "register values"() -> (w582:u16[])
            n290 = Index Array(array=w582, index=1 ("索引")) -> (element=w580:u16)
            n291 = Index Array(array=w578, index=0 ("索引")) -> (element=w577:u16)
          }
          frame "氨氮" {
            n292 = global read "全局1.vi" "读取试剂余量的值"() -> (w584:u16[])
            n293 = global read "全局1.vi" "register values"() -> (w588:u16[])
            n294 = Index Array(array=w588, index=2 ("索引")) -> (element=w586:u16)
            n295 = Index Array(array=w584, index=1 ("索引")) -> (element=w583:u16)
          }
          frame "总磷" {
            n296 = global read "全局1.vi" "读取试剂余量的值"() -> (w590:u16[])
            n297 = global read "全局1.vi" "register values"() -> (w594:u16[])
            n298 = Index Array(array=w594, index=3 ("索引")) -> (element=w592:u16)
            n299 = Index Array(array=w590, index=2 ("索引")) -> (element=w589:u16)
          }
          frame "总氮" {
            n300 = global read "全局1.vi" "读取试剂余量的值"() -> (w596:u16[])
            n301 = global read "全局1.vi" "register values"() -> (w600:u16[])
            n302 = Index Array(array=w600, index=4 ("索引")) -> (element=w598:u16)
            n303 = Index Array(array=w596, index=3 ("索引")) -> (element=w595:u16)
          }
          frame "CODCr" {
            n304 = global read "全局1.vi" "读取试剂余量的值"() -> (w602:u16[])
            n305 = global read "全局1.vi" "register values"() -> (w606:u16[])
            n306 = Index Array(array=w606, index=5 ("索引")) -> (element=w604:u16)
            n307 = Index Array(array=w602, index=4 ("索引")) -> (element=w601:u16)
          }
        }
        n308 = global read "全局 小时数据发送次数.vi" "小时数据发送次数"() -> (w557:i32)
        n309 = Unbundle By Name(w562) -> ("藻密度"=w561:string)
        n310 = Equal?(x=w559, y=w561) -> (x = y?=w549:bool)
        n311 = Index Array(array=w556, index (row)=w557) -> (element=w555:string[])  [unwired: 1 in]
        n312 = Select(t="w00000", s=w549, f=w559) -> (s? t:f=w558:string)
        n313 = Index Array(array=w555, index #1=0 ("索引"), index #2=2 ("索引")) -> (element #1=w536:string, element #2=w568:string)
        n314 = Empty String/Path?(string/path=w536) -> (empty?=w567:bool)
        n315 = Select(t="i22001", s=w549, f="i12001") -> (s? t:f=w548:string)
        n316 = Select(t="i22003", s=w549, f="i12031") -> (s? t:f=w547:string)
        n317 = Number To Decimal String(number=w552) -> (decimal integer string=w553:string)  [unwired: 1 in]
        n318 = Number To Decimal String(number=w537) -> (decimal integer string=w538:string)  [unwired: 1 in]
        n319 = case shown="False" w567 {
          tunnel: [w615 _] -> w544
          tunnel: w568 -> [w612 _]
          tunnel: w558 -> [w610 _]
          tunnel: w553 -> [w608 _]
          tunnel: w548 -> [w609 _]
          tunnel: w547 -> [w613 _]
          tunnel: w538 -> [w607 _]
          frame False {
            n320 = call "告警信息文本转换为协议i12031值.vi"("字符串"=w612) -> ("十进制整型字符串"=w611:string)  [unwired: 10 in]
            n321 = Format Into String(format string="PolId=%s,%s-Info=%s,i12002-Info=0,i12003-Info=%s,%s-Info=%s;" ("格式字符串"), w610, w609, w608, w607, w613, w611) -> (resulting string=w615:string)  [unwired: 2 in, 1 out]
          }
          frame True {
          }
        }
        n322 = Empty String/Path?(string/path=w544) -> (empty?=w543:bool)
        n323 = Concatenate Strings(w540, w544) -> (w546:string)
        n324 = Not(x=w543) -> (.not. x?=w542:bool)
        n325 = And(x=w539, y=w542) -> (x .and. y?=w541:bool)
        n326 = case shown="True" w541 {
          tunnel: w536 -> [_ w572]
          tunnel: w546 -> [w569 w571]
          tunnel: [w569 w570] -> w545
          frame False {
          }
          frame True {
            n327 = call "规范时间戳.vi"("字符串"=w572) -> ("result string"=w574:string)  [unwired: 10 in]
            n328 = Format Into String(format string="DataTime=%s;%s", w574, w571) -> (resulting string=w570:string)  [unwired: 2 in, 1 out]
          }
        }
      }
    }
  }
  "字符串" <- w25
